vi "SplitStrings.vi"(9 "Delimiter String":string, 10 "Input String":string) -> (2 "Strings":string[](array[string]))   [LabVIEW 2015, in "ProdigyRemoteControl.lvlib"]
uses:
  ProdigyRemoteControl.lvlib
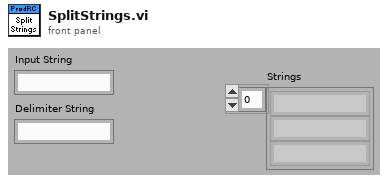
[diagram p1: front panel]
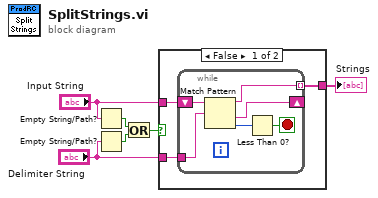
[diagram p0: block diagram]
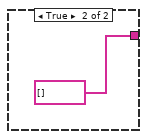
[diagram p2: hidden frame]
diagram:
  n1 = Empty String/Path?(string/path="Input String") -> (empty?=w5:bool)
  n2 = Empty String/Path?(string/path="Delimiter String") -> (empty?=w6:bool)
  n3 = Or(x=w5, y=w6) -> (x .or. y?=w4:bool)
  n4 = case shown="False" w4 {
    tunnel: "Input String" -> [w9 _]
    tunnel: "Delimiter String" -> [w8 _]
    tunnel: [w7 string[] [] ("Strings")] -> w1
    frame False {
      n5 = while {
        shift-right: [w10] -> _
        shift-left: w9 -> [w15]
        tunnel: w8 -> [w14]
        tunnel: [w11] -> w7 mode=indexing
        stop <- w12 stop-if-true
        n6 = Match Pattern(string=w15, regular expression=w14) -> (before substring=w11:string, after substring=w10:string, offset past match=w13:i32)  [unwired: 1 in, 1 out]
        n7 = Less Than 0?(x=w13) -> (x < 0?=w12:bool)
      }
    }
    frame True {
    }
  }
  "Strings" <- w1
